vi "LvDatatypeToImageType_U16.vi"(9 "error in":errorcluster, 11 "Numeric":u16) -> (1 "error out":errorcluster, 2 "Image Type":T1, 3 "Numeric out":u16)   [LabVIEW 2020, in "OpenLvVision_OpenCv.lvlib"]
doc: "converts 2d array to image format"
uses:
  OpenLvVision_OpenCv.lvlib
  <vilib>/OpenLvVision/OpenLvVision_Image/Management/TypeDef/OLV ImageType.ctl
  <vilib>/OpenLvVision/OpenLvVision_Image/Management/OLV Management.lvlib
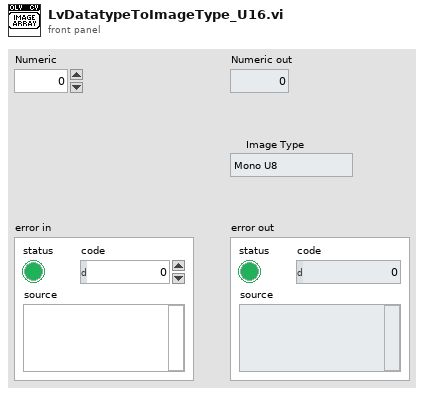
[diagram p1: front panel]
types:
  T1 = typedef "OLV OpenLvVision_Image.lvlib/OLV Management.lvlib/OLV ImageType.ctl" = enum16{"Mono U8", "Mono U16", "Mono I16", "Mono SGL", "Color U32", "Color U64", "Complex CSG"}
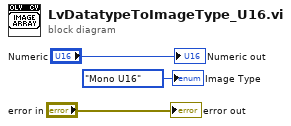
[diagram p0: block diagram]
diagram:
  "Image Type" <- OLV_ImageType."Mono U16" ("Image Type")
  "Numeric out" <- "Numeric"
  "error out" <- "error in"
